vi "is_valid.vi"(11 "obj in":refnum<class "RequestBuilder.lvclass">) -> (2 "valid-ref?":bool)   [LabVIEW 2020, in "reqwest.lvlib" / "RequestBuilder.lvclass"]
uses:
  RequestBuilder.lvclass
  RequestBuilder.lvclass/RequestBuilder.ctl
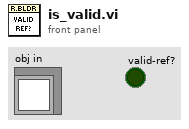
[diagram p1: front panel]
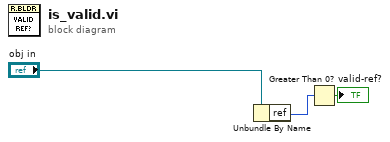
[diagram p0: block diagram]
diagram:
  n1 = Unbundle By Name("obj in") -> ("ref"=w2:u64)
  n2 = Greater Than 0?(x=w2) -> (x > 0?=→"valid-ref?":bool)
